vi "INST_PS_CONFIG_OUTPUT.vi"(0 "VISA session":refnum<visa-resource-name>="TCPIP0::169.254.70.130::inst0::INSTR", 1 "SEL_PS":string(combo)="PS1", 2 "RO(T)":bool, 11 "error in (no error)":errorcluster, 12 "Instrument Select (Output 1)":string(combo)="1", 13 "Enable Output (False)":bool, 14 "Use OPC(T)":bool) -> (4 "dup VISA session":refnum<visa-resource-name>, 8 "read_out_stat_on(t)":bool[](array[boolean]), 15 "error out":errorcluster)   [LabVIEW 2018]
doc: "This VI configures the DC voltage level the power supply attempts to generate.\n\nVer 3.0.0 supports the E36xx Model and The 6634B based on the GPIB address of idtATE [10-12]"
uses:
  Initialize References/Station References Global.vi
panel:
  out "PSn Model":string
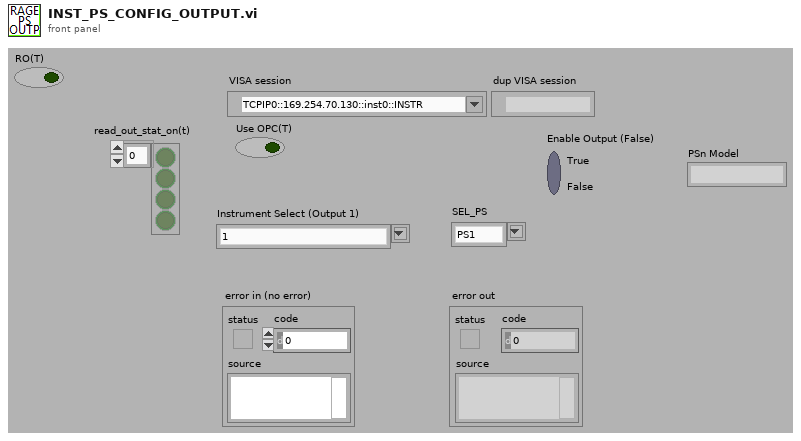
[diagram p1: front panel]
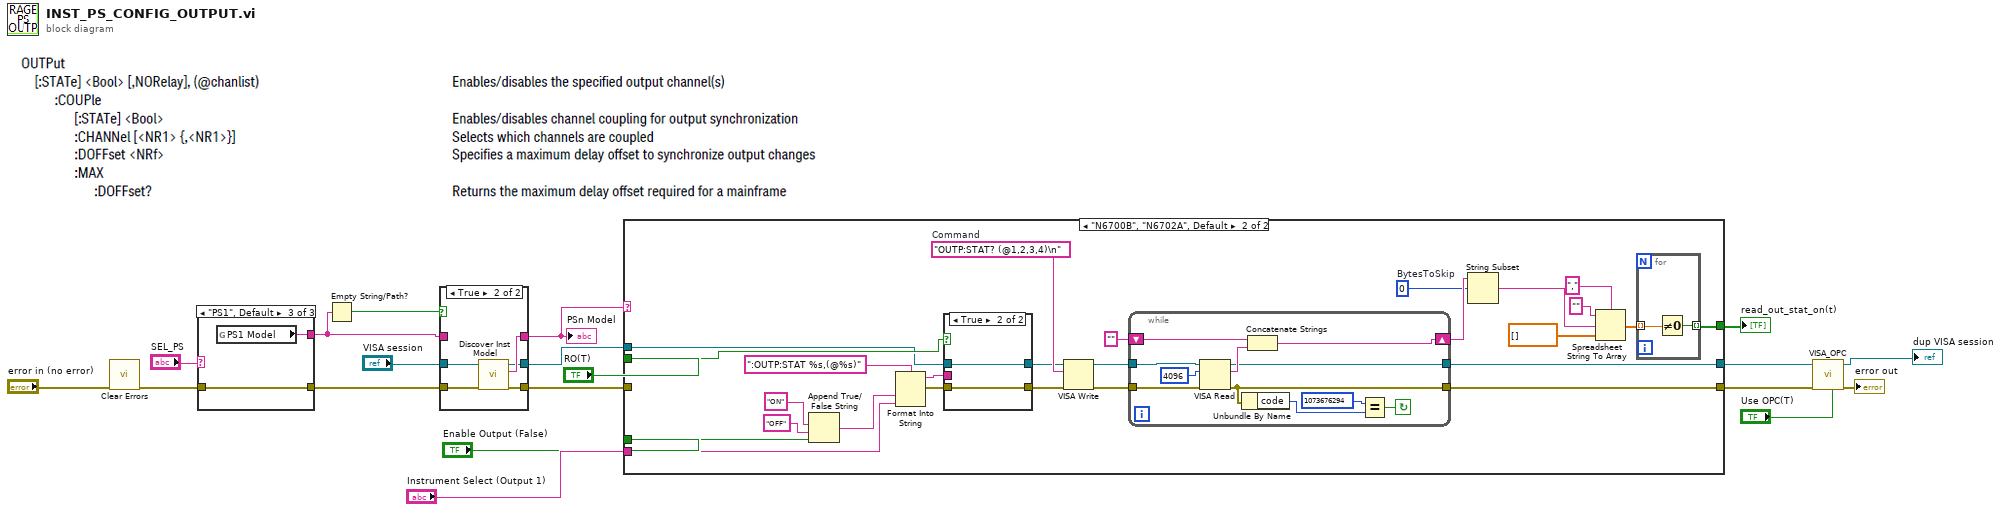
[diagram p0: block diagram]
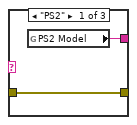
[diagram p3: hidden frame]
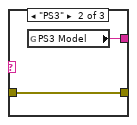
[diagram p4: hidden frame]
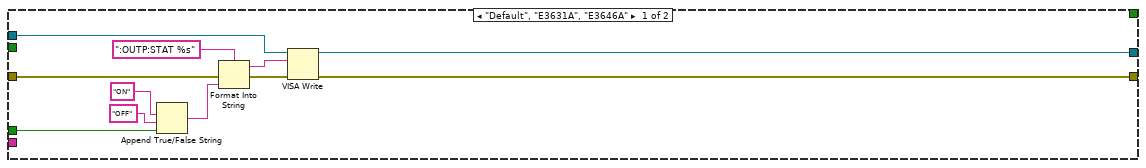
[diagram p5: hidden frame]
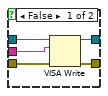
[diagram p6: hidden frame]
diagram:
  n1 = call <vilib>:"Clear Errors.vi"("error in (no error)"="error in (no error)") -> ("error out"=w6:errorcluster)  [unwired: 5 in, 1 out]
  n2 = case shown="\"PS1\", Default" "SEL_PS" {
    tunnel: [w21 w23 w25] -> w9
    tunnel: w6 -> [w20 w22 w24]
    tunnel: [w20 w22 w24] -> w12
    frame "PS2" {
      n3 = global read "Station References Global.vi" "PS2 Model"() -> (w21:string)
    }
    frame "PS3" {
      n4 = global read "Station References Global.vi" "PS3 Model"() -> (w23:string)
    }
    frame "PS1", Default {
      n5 = global read "Station References Global.vi" "PS1 Model"() -> (w25:string)
    }
  }
  n6 = Empty String/Path?(string/path=w9) -> (empty?=w8:bool)
  n7 = case shown="True" w8 {
    tunnel: [w27 w33] -> w13
    tunnel: "VISA session" -> [w28 w32]
    tunnel: [w28 w31] -> w5
    tunnel: w9 -> [w27 _]
    tunnel: w12 -> [w26 w30]
    tunnel: [w26 w29] -> w11
    frame False {
    }
    frame True {
      n8 = call "Discover Inst Model.vi"("error in"=w30, "Session In"=w32) -> ("error out"=w29:errorcluster, "Model #"=w33:string, "Session Out"=w31:refnum<visa-resource-name>)  [unwired: 7 in]
    }
  }
  "PSn Model" <- w13
  n9 = case shown="\"N6700B\", \"N6702A\", Default" w13 {
    tunnel: "Instrument Select (Output 1)" -> [_ w65]
    tunnel: w11 -> [w39 _]
    tunnel: "Enable Output (False)" -> [w40 w69]
    tunnel: [w36 w52] -> w3
    tunnel: w5 -> [w35 w46]
    tunnel: [w34 w53] -> w4
    tunnel: "RO(T)" -> [_ w56]
    tunnel: [_ w48] -> w1
    frame "Default", "E3631A", "E3646A" {
      n10 = Append True/False String(1:w40, 2:"OFF", 3:"ON") -> (0:w44:string)  [unwired: 1 in]
      n11 = Format Into String(format string=":OUTP:STAT %s", error in=w39, w44) -> (resulting string=w37:string, error out=w38:errorcluster)  [unwired: 1 in]
      n12 = VISA Write(VISA resource name=w35, write buffer=w37, error in (no error)=w38) -> (VISA resource name out=w34:refnum<visa-resource-name>, error out=w36:errorcluster)  [unwired: 1 out]
    }
    frame "N6700B", "N6702A", Default {
      w61 = 0  # BytesToSkip
      w59 = "OUTP:STAT? (@1,2,3,4)\n"  # Command
      n13 = Append True/False String(1:w69, 2:"OFF", 3:"ON") -> (0:w70:string)  [unwired: 1 in]
      n14 = Format Into String(format string=":OUTP:STAT %s,(@%s)", w70, w65) -> (resulting string=w57:string, error out=w55:errorcluster)  [unwired: 2 in]
      n15 = case shown="True" w56 {
        tunnel: w57 -> [w77 _]
        tunnel: [w76 w78] -> w45
        tunnel: w55 -> [w75 w79]
        tunnel: [w74 w79] -> w54
        tunnel: w46 -> [w73 w78]
        frame False {
          n16 = VISA Write(VISA resource name=w73, write buffer=w77, error in (no error)=w75) -> (VISA resource name out=w76:refnum<visa-resource-name>, error out=w74:errorcluster)  [unwired: 1 out]
        }
        frame True {
        }
      }
      n17 = VISA Write(VISA resource name=w45, write buffer=w59, error in (no error)=w54) -> (VISA resource name out=w64:refnum<visa-resource-name>, error out=w63:errorcluster)  [unwired: 1 out]
      n18 = while {
        tunnel: w64 -> [w87]
        shift-right: [w81] -> w62
        shift-left: "" -> [w86]
        tunnel: w63 -> [w84]
        tunnel: [w83] -> w52
        tunnel: [w80] -> w53
        stop <- w82 continue-if-true
        n19 = VISA Read(VISA resource name=w87, byte count=u32 4096 ("byte count (0)"), error in (no error)=w84) -> (VISA resource name out=w80:refnum<visa-resource-name>, read buffer=w85:string, error out=w83:errorcluster)  [unwired: 1 out]
        n20 = Unbundle By Name(w83) -> ("code"=w89:i32)
        n21 = Concatenate Strings(w86, w85) -> (w81:string)
        n22 = Equal?(x=1073676294, y=w89) -> (x = y?=w82:bool)
      }
      n23 = String Subset(string=w62, offset (0)=w61) -> (substring=w58:string)  [unwired: 1 out]
      n24 = Spreadsheet String To Array(delimiter (Tab)=",", format string="", spreadsheet string=w58, array type (2D Dbl)=dbl[] []) -> (array=w49:dbl[])
      n25 = for {
        tunnel: w49 -> [w72] mode=indexing
        tunnel: [w71] -> w48 mode=indexing
        n26 = Not Equal To 0?(x=w72) -> (x != 0?=w71:bool)
      }
    }
  }
  "read_out_stat_on(t)" <- w1
  n27 = call "VISA_OPC.vi"("OPC(T)"="Use OPC(T)", "error in"=w3, "Session In"=w4) -> ("error out"=→"error out":errorcluster, "Session Out"=→"dup VISA session":refnum<visa-resource-name>)  [unwired: 6 in, 1 out]
